vi "configureDigitalOutput.vi"(8 "error in (no error)":errorcluster, 9 "DigitalOutput":refnum<class "DigitalOutput.lvclass">, 10 "deviceName":string, 11 "BECHWCBasic in":refnum<class "BECHWCBasic.lvclass">) -> (0 "error out":errorcluster, 3 "BECHWCBasic out":refnum<class "BECHWCBasic.lvclass">)   [LabVIEW 2009, in "Hardware.lvlib" / "HWControllers.lvlib" / "BECHWCBasic.lvclass"]
doc: "Configure the digital output channels of a device"
uses:
  BECHWCBasic.lvclass
  Channels/Digital/DigitalOutput.lvclass
  BECHWCBasic.lvclass/BECHWCBasic.ctl
  HWController.lvclass
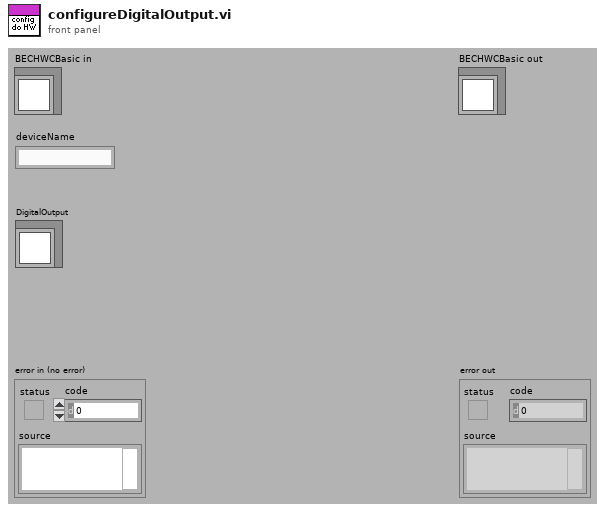
[diagram p1: front panel]
types:
  T1 = cluster{"Master Clock source":string, "Master Clock rate":dbl, "Start trigger line":string, "Scan rate":dbl, "Stop trigger line":string, "Sample Number":dbl}
  T2 = cluster{"Timestamps ms":dbl[], "DataPerChannel":dbl[][]}
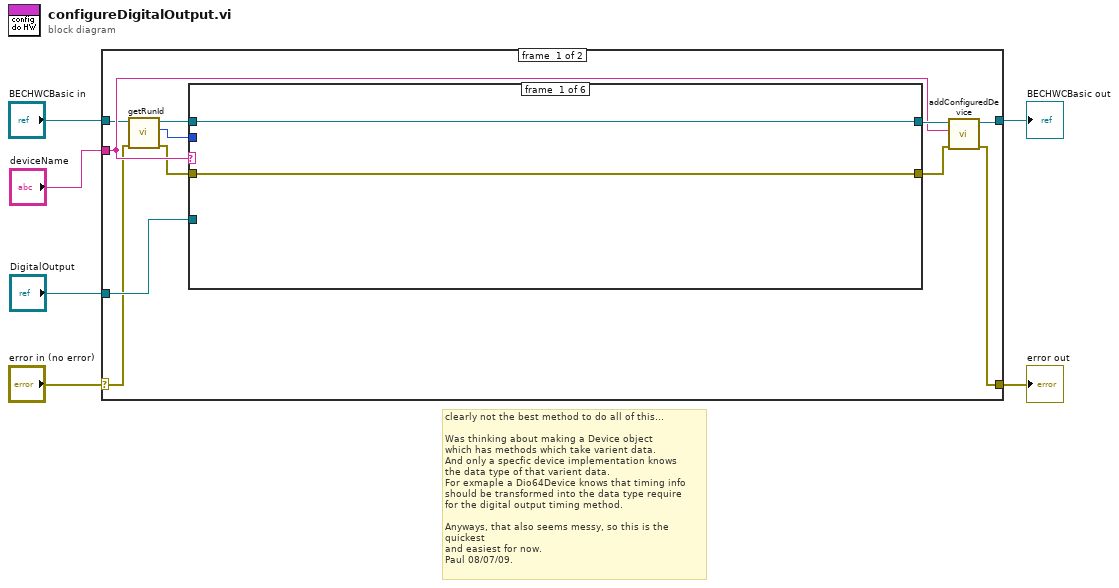
[diagram p0: block diagram]
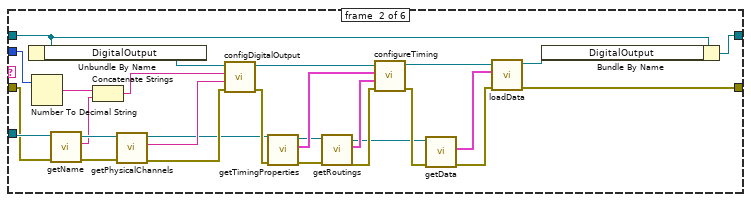
[diagram p2: hidden frame]
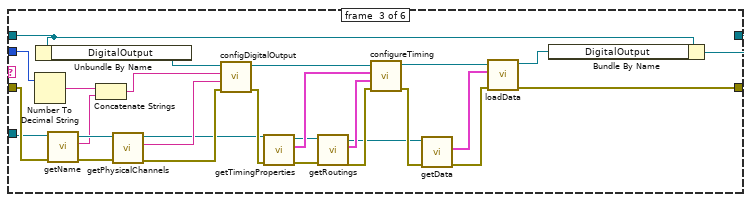
[diagram p3: hidden frame]
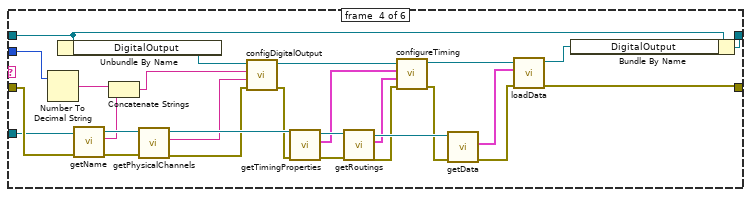
[diagram p4: hidden frame]
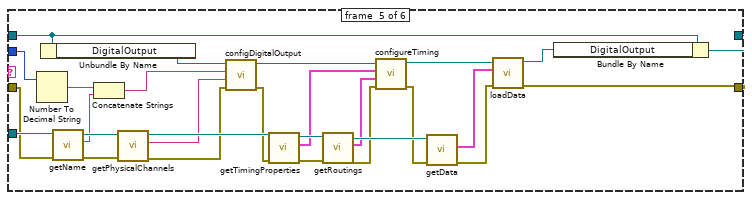
[diagram p5: hidden frame]
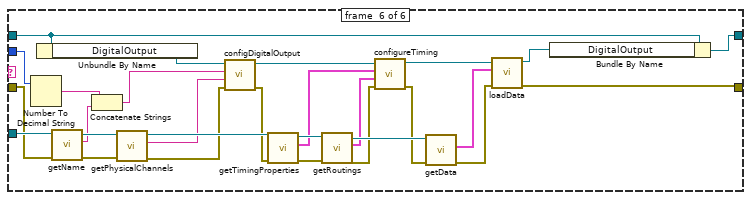
[diagram p6: hidden frame]
diagram:
  # "clearly not the best method to do all of this...\n \nWas thinking about making a Device object\nwhich has methods which take varient data.\nAnd only a specfic device implementation knows\nthe data type of that varient data. \nFor exmaple a Dio64Device knows that timing info\nshould be transformed into the data type require\nfor the digital output timing method.\n\nAnyways, that also seems messy, so this is the quickest\nand easiest for now.\nPaul 08/07/09."
  n1 = case shown="No Error" "error in (no error)" {
    selector: "error in (no error)" -> [w8 w161]
    tunnel: [w13 w161] -> w5
    tunnel: [w15 w160] -> w3
    tunnel: "BECHWCBasic in" -> [w11 w160]
    tunnel: "deviceName" -> [w12 _]
    tunnel: "DigitalOutput" -> [w17 _]
    frame #0 {
      n2 = call "getRunId.vi"("error in (no error)"=w8, "HWController in"=w11) -> ("error out"=w7:errorcluster, "Numeric"=w9:i32, "HWController out"=w10:refnum<class "BECHWCBasic.lvclass">)  [unwired: 7 in]
      n3 = case shown="\"Dio64\"" w12 {
        tunnel: w10 -> [w19 w28 w56 w85 w112 w138]
        tunnel: [w19 w27 w55 w84 w108 w137] -> w16
        tunnel: w7 -> [w18 w24 w53 w82 w110 w151]
        tunnel: [w18 w26 w54 w83 w109 w139] -> w14
        tunnel: w17 -> [_ w25 w52 w81 w111 w152]
        tunnel: w9 -> [_ w23 w50 w77 w106 w134]
        frame #0 {
        }
        frame #1 {
          n4 = Unbundle By Name(w28) -> ("DigitalOutput"=w36:refnum<class "DigitalOutput.lvclass">)
          n5 = Number To Decimal String(number=w23) -> (decimal integer string=w22:string)  [unwired: 1 in]
          n6 = call-dynamic "getName.vi"("error in (no error)"=w24, "DigitalOutput.lvclass in"=w25) -> ("error out"=w31:errorcluster, "name"=w21:string, "DigitalOutput.lvclass out"=w30:refnum<class "DigitalOutput.lvclass">)  [unwired: 7 in]
          n7 = Concatenate Strings(w22, w21) -> (w20:string)
          n8 = call-dynamic "getPhysicalChannels.vi"("error in (no error)"=w31, "DigitalOutput.lvclass in"=w30) -> ("error out"=w38:errorcluster, "Physical Channels"=w37:string, "DigitalOutput.lvclass out"=w32:refnum<class "DigitalOutput.lvclass">)  [unwired: 7 in]
          n9 = call-dynamic "configDigitalOutput.vi"("error in (no error)"=w38, "Physical Channels"=w37, "name"=w20, "DigitalOutput in"=w36) -> ("error out"=w39:errorcluster, "DigitalOutput out"=w40:refnum<class "DigitalOutput.lvclass">)  [unwired: 6 in]
          n10 = call-dynamic "getTimingProperties.vi"("error in (no error)"=w39, "DigitalOutput.lvclass in"=w32) -> ("error out"=w34:errorcluster, "Timing"=w41:T1, "DigitalOutput.lvclass out"=w33:refnum<class "DigitalOutput.lvclass">)  [unwired: 7 in]
          n11 = call-dynamic "getRoutings.vi"("error in (no error)"=w34, "DigitalOutput.lvclass in"=w33) -> ("error out"=w43:errorcluster, "Routings"=w42:cluster{"Master Clock Route":string[]}, "DigitalOutput.lvclass out"=w35:refnum<class "DigitalOutput.lvclass">)  [unwired: 7 in]
          n12 = call-dynamic "configureTiming.vi"("error in (no error)"=w43, "Routings"=w42, "Timing"=w41, "DigitalOutput in"=w40) -> ("error out"=w44:errorcluster, "DigitalOutput out"=w29:refnum<class "DigitalOutput.lvclass">)  [unwired: 6 in]
          n13 = call-dynamic "getData.vi"("error in (no error)"=w44, "DigitalOutput.lvclass in"=w35) -> ("error out"=w46:errorcluster, "Data"=w45:T2)  [unwired: 7 in, 1 out]
          n14 = call-dynamic "loadData.vi"("error in (no error)"=w46, "Data"=w45, "DigitalOutput in"=w29) -> ("error out"=w26:errorcluster, "DigitalOutput out"=w47:refnum<class "DigitalOutput.lvclass">)  [unwired: 7 in]
          n15 = Bundle By Name(cluster=w28, "DigitalOutput"=w47) -> (w27:refnum<class "BECHWCBasic.lvclass">)
        }
        frame #2 {
          n16 = Number To Decimal String(number=w50) -> (decimal integer string=w51:string)  [unwired: 1 in]
          n17 = Unbundle By Name(w56) -> ("DigitalOutput"=w64:refnum<class "DigitalOutput.lvclass">)
          n18 = call-dynamic "getName.vi"("error in (no error)"=w53, "DigitalOutput.lvclass in"=w52) -> ("error out"=w59:errorcluster, "name"=w49:string, "DigitalOutput.lvclass out"=w58:refnum<class "DigitalOutput.lvclass">)  [unwired: 7 in]
          n19 = Concatenate Strings(w51, w49) -> (w48:string)
          n20 = call-dynamic "getPhysicalChannels.vi"("error in (no error)"=w59, "DigitalOutput.lvclass in"=w58) -> ("error out"=w66:errorcluster, "Physical Channels"=w65:string, "DigitalOutput.lvclass out"=w60:refnum<class "DigitalOutput.lvclass">)  [unwired: 7 in]
          n21 = call-dynamic "configDigitalOutput.vi"("error in (no error)"=w66, "Physical Channels"=w65, "name"=w48, "DigitalOutput in"=w64) -> ("error out"=w67:errorcluster, "DigitalOutput out"=w68:refnum<class "DigitalOutput.lvclass">)  [unwired: 6 in]
          n22 = call-dynamic "getTimingProperties.vi"("error in (no error)"=w67, "DigitalOutput.lvclass in"=w60) -> ("error out"=w62:errorcluster, "Timing"=w69:T1, "DigitalOutput.lvclass out"=w61:refnum<class "DigitalOutput.lvclass">)  [unwired: 7 in]
          n23 = call-dynamic "getRoutings.vi"("error in (no error)"=w62, "DigitalOutput.lvclass in"=w61) -> ("error out"=w71:errorcluster, "Routings"=w70:cluster{"Master Clock Route":string[]}, "DigitalOutput.lvclass out"=w63:refnum<class "DigitalOutput.lvclass">)  [unwired: 7 in]
          n24 = call-dynamic "configureTiming.vi"("error in (no error)"=w71, "Routings"=w70, "Timing"=w69, "DigitalOutput in"=w68) -> ("error out"=w72:errorcluster, "DigitalOutput out"=w57:refnum<class "DigitalOutput.lvclass">)  [unwired: 6 in]
          n25 = call-dynamic "getData.vi"("error in (no error)"=w72, "DigitalOutput.lvclass in"=w63) -> ("error out"=w74:errorcluster, "Data"=w73:T2)  [unwired: 7 in, 1 out]
          n26 = call-dynamic "loadData.vi"("error in (no error)"=w74, "Data"=w73, "DigitalOutput in"=w57) -> ("error out"=w54:errorcluster, "DigitalOutput out"=w75:refnum<class "DigitalOutput.lvclass">)  [unwired: 7 in]
          n27 = Bundle By Name(cluster=w56, "DigitalOutput"=w75) -> (w55:refnum<class "BECHWCBasic.lvclass">)
        }
        frame #3 {
          n28 = Number To Decimal String(number=w77) -> (decimal integer string=w80:string)  [unwired: 1 in]
          n29 = Unbundle By Name(w85) -> ("DigitalOutput"=w96:refnum<class "DigitalOutput.lvclass">)
          n30 = call-dynamic "getName.vi"("error in (no error)"=w82, "DigitalOutput.lvclass in"=w81) -> ("error out"=w101:errorcluster, "name"=w79:string, "DigitalOutput.lvclass out"=w102:refnum<class "DigitalOutput.lvclass">)  [unwired: 7 in]
          n31 = Concatenate Strings(w80, w79) -> (w78:string)
          n32 = call-dynamic "getPhysicalChannels.vi"("error in (no error)"=w101, "DigitalOutput.lvclass in"=w102) -> ("error out"=w94:errorcluster, "Physical Channels"=w95:string, "DigitalOutput.lvclass out"=w100:refnum<class "DigitalOutput.lvclass">)  [unwired: 7 in]
          n33 = call-dynamic "configDigitalOutput.vi"("error in (no error)"=w94, "Physical Channels"=w95, "name"=w78, "DigitalOutput in"=w96) -> ("error out"=w93:errorcluster, "DigitalOutput out"=w92:refnum<class "DigitalOutput.lvclass">)  [unwired: 6 in]
          n34 = call-dynamic "getTimingProperties.vi"("error in (no error)"=w93, "DigitalOutput.lvclass in"=w100) -> ("error out"=w98:errorcluster, "Timing"=w76:T1, "DigitalOutput.lvclass out"=w99:refnum<class "DigitalOutput.lvclass">)  [unwired: 7 in]
          n35 = call-dynamic "getRoutings.vi"("error in (no error)"=w98, "DigitalOutput.lvclass in"=w99) -> ("error out"=w90:errorcluster, "Routings"=w91:cluster{"Master Clock Route":string[]}, "DigitalOutput.lvclass out"=w97:refnum<class "DigitalOutput.lvclass">)  [unwired: 7 in]
          n36 = call-dynamic "configureTiming.vi"("error in (no error)"=w90, "Routings"=w91, "Timing"=w76, "DigitalOutput in"=w92) -> ("error out"=w89:errorcluster, "DigitalOutput out"=w103:refnum<class "DigitalOutput.lvclass">)  [unwired: 6 in]
          n37 = call-dynamic "getData.vi"("error in (no error)"=w89, "DigitalOutput.lvclass in"=w97) -> ("error out"=w87:errorcluster, "Data"=w88:T2)  [unwired: 7 in, 1 out]
          n38 = call-dynamic "loadData.vi"("error in (no error)"=w87, "Data"=w88, "DigitalOutput in"=w103) -> ("error out"=w83:errorcluster, "DigitalOutput out"=w86:refnum<class "DigitalOutput.lvclass">)  [unwired: 7 in]
          n39 = Bundle By Name(cluster=w85, "DigitalOutput"=w86) -> (w84:refnum<class "BECHWCBasic.lvclass">)
        }
        frame #4 {
          n40 = Number To Decimal String(number=w106) -> (decimal integer string=w107:string)  [unwired: 1 in]
          n41 = Unbundle By Name(w112) -> ("DigitalOutput"=w124:refnum<class "DigitalOutput.lvclass">)
          n42 = call-dynamic "getName.vi"("error in (no error)"=w110, "DigitalOutput.lvclass in"=w111) -> ("error out"=w129:errorcluster, "name"=w105:string, "DigitalOutput.lvclass out"=w130:refnum<class "DigitalOutput.lvclass">)  [unwired: 7 in]
          n43 = Concatenate Strings(w107, w105) -> (w104:string)
          n44 = call-dynamic "getPhysicalChannels.vi"("error in (no error)"=w129, "DigitalOutput.lvclass in"=w130) -> ("error out"=w122:errorcluster, "Physical Channels"=w123:string, "DigitalOutput.lvclass out"=w128:refnum<class "DigitalOutput.lvclass">)  [unwired: 7 in]
          n45 = call-dynamic "configDigitalOutput.vi"("error in (no error)"=w122, "Physical Channels"=w123, "name"=w104, "DigitalOutput in"=w124) -> ("error out"=w121:errorcluster, "DigitalOutput out"=w120:refnum<class "DigitalOutput.lvclass">)  [unwired: 6 in]
          n46 = call-dynamic "getTimingProperties.vi"("error in (no error)"=w121, "DigitalOutput.lvclass in"=w128) -> ("error out"=w126:errorcluster, "Timing"=w119:T1, "DigitalOutput.lvclass out"=w127:refnum<class "DigitalOutput.lvclass">)  [unwired: 7 in]
          n47 = call-dynamic "getRoutings.vi"("error in (no error)"=w126, "DigitalOutput.lvclass in"=w127) -> ("error out"=w117:errorcluster, "Routings"=w118:cluster{"Master Clock Route":string[]}, "DigitalOutput.lvclass out"=w125:refnum<class "DigitalOutput.lvclass">)  [unwired: 7 in]
          n48 = call-dynamic "configureTiming.vi"("error in (no error)"=w117, "Routings"=w118, "Timing"=w119, "DigitalOutput in"=w120) -> ("error out"=w116:errorcluster, "DigitalOutput out"=w131:refnum<class "DigitalOutput.lvclass">)  [unwired: 6 in]
          n49 = call-dynamic "getData.vi"("error in (no error)"=w116, "DigitalOutput.lvclass in"=w125) -> ("error out"=w114:errorcluster, "Data"=w115:T2)  [unwired: 7 in, 1 out]
          n50 = call-dynamic "loadData.vi"("error in (no error)"=w114, "Data"=w115, "DigitalOutput in"=w131) -> ("error out"=w109:errorcluster, "DigitalOutput out"=w113:refnum<class "DigitalOutput.lvclass">)  [unwired: 7 in]
          n51 = Bundle By Name(cluster=w112, "DigitalOutput"=w113) -> (w108:refnum<class "BECHWCBasic.lvclass">)
        }
        frame #5 {
          n52 = Number To Decimal String(number=w134) -> (decimal integer string=w135:string)  [unwired: 1 in]
          n53 = Unbundle By Name(w138) -> ("DigitalOutput"=w150:refnum<class "DigitalOutput.lvclass">)
          n54 = call-dynamic "getName.vi"("error in (no error)"=w151, "DigitalOutput.lvclass in"=w152) -> ("error out"=w157:errorcluster, "name"=w133:string, "DigitalOutput.lvclass out"=w158:refnum<class "DigitalOutput.lvclass">)  [unwired: 7 in]
          n55 = Concatenate Strings(w135, w133) -> (w132:string)
          n56 = call-dynamic "getPhysicalChannels.vi"("error in (no error)"=w157, "DigitalOutput.lvclass in"=w158) -> ("error out"=w148:errorcluster, "Physical Channels"=w149:string, "DigitalOutput.lvclass out"=w156:refnum<class "DigitalOutput.lvclass">)  [unwired: 7 in]
          n57 = call-dynamic "configDigitalOutput.vi"("error in (no error)"=w148, "Physical Channels"=w149, "name"=w132, "DigitalOutput in"=w150) -> ("error out"=w147:errorcluster, "DigitalOutput out"=w146:refnum<class "DigitalOutput.lvclass">)  [unwired: 6 in]
          n58 = call-dynamic "getTimingProperties.vi"("error in (no error)"=w147, "DigitalOutput.lvclass in"=w156) -> ("error out"=w154:errorcluster, "Timing"=w145:T1, "DigitalOutput.lvclass out"=w155:refnum<class "DigitalOutput.lvclass">)  [unwired: 7 in]
          n59 = call-dynamic "getRoutings.vi"("error in (no error)"=w154, "DigitalOutput.lvclass in"=w155) -> ("error out"=w143:errorcluster, "Routings"=w144:cluster{"Master Clock Route":string[]}, "DigitalOutput.lvclass out"=w153:refnum<class "DigitalOutput.lvclass">)  [unwired: 7 in]
          n60 = call-dynamic "configureTiming.vi"("error in (no error)"=w143, "Routings"=w144, "Timing"=w145, "DigitalOutput in"=w146) -> ("error out"=w142:errorcluster, "DigitalOutput out"=w159:refnum<class "DigitalOutput.lvclass">)  [unwired: 6 in]
          n61 = call-dynamic "getData.vi"("error in (no error)"=w142, "DigitalOutput.lvclass in"=w153) -> ("error out"=w140:errorcluster, "Data"=w141:T2)  [unwired: 7 in, 1 out]
          n62 = call-dynamic "loadData.vi"("error in (no error)"=w140, "Data"=w141, "DigitalOutput in"=w159) -> ("error out"=w139:errorcluster, "DigitalOutput out"=w136:refnum<class "DigitalOutput.lvclass">)  [unwired: 7 in]
          n63 = Bundle By Name(cluster=w138, "DigitalOutput"=w136) -> (w137:refnum<class "BECHWCBasic.lvclass">)
        }
      }
      n64 = call "addConfiguredDevice.vi"("error in (no error)"=w14, "deviceName"=w12, "HWController in"=w16) -> ("error out"=w13:errorcluster, "HWController out"=w15:refnum<class "BECHWCBasic.lvclass">)  [unwired: 7 in]
    }
    frame #1 {
    }
  }
  "error out" <- w5
  "BECHWCBasic out" <- w3
